vi "5_ASK.vi"() -> ()   [LabVIEW 2026]
uses:
  <vilib>/Analysis/NI_AALPro.lvlib
panel:
  out "Waveform Chart 2":dbl[](graph)
  out "Array":bool[](array[boolean])
  out "Waveform Chart":dbl[](graph)
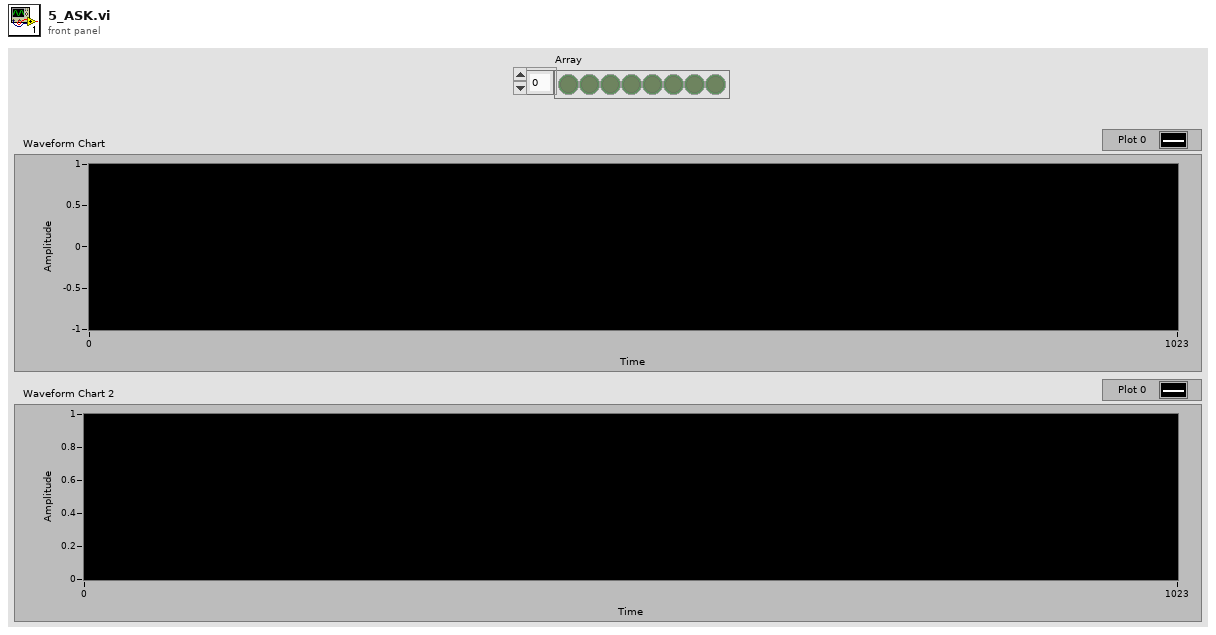
[diagram p1: front panel]
types:
  T1 = enum16{"sine", "cosine", "triangle", "square", "sawtooth", "increasing ramp", "decreasing ramp"}
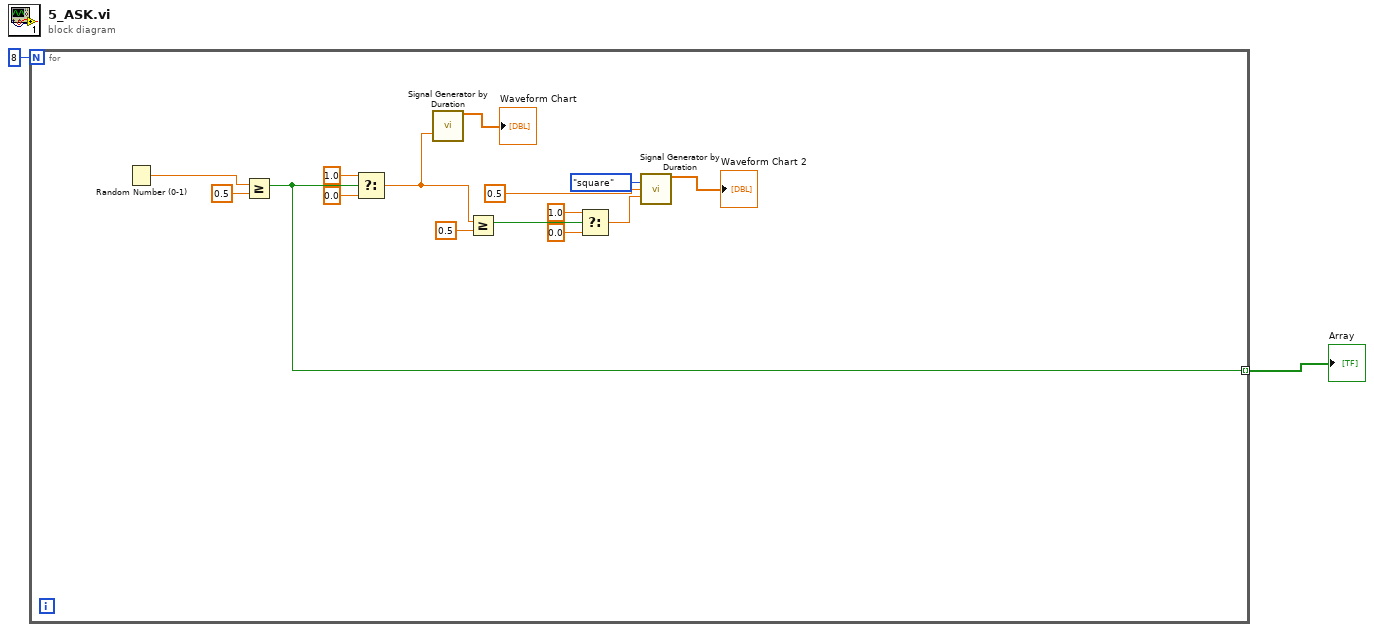
[diagram p0: block diagram]
diagram:
  n1 = for {
    N: 8 -> [_]
    tunnel: [w12] -> w1 mode=indexing
    n2 = Random Number (0-1)() -> (number: 0 to 1=w17:dbl)
    n3 = Greater Or Equal?(x=w17, y=0.5) -> (x >= y?=w12:bool)
    n4 = Select(t=1.0, s=w12, f=0.0) -> (s? t:f=w7:dbl)
    n5 = call <vilib>:"Signal Generator by Duration.vi"("amplitude"=w7) -> ("signal"=→"Waveform Chart":dbl[])  [unwired: 11 in, 3 out]
    n6 = Greater Or Equal?(x=w7, y=0.5) -> (x >= y?=w8:bool)
    n7 = Select(t=1.0, s=w8, f=0.0) -> (s? t:f=w6:dbl)
    n8 = call <vilib>:"Signal Generator by Duration.vi"("signal type"=T1."square", "frequency"=0.5, "amplitude"=w6) -> ("signal"=→"Waveform Chart 2":dbl[])  [unwired: 9 in, 3 out]
  }
  "Array" <- w1
